vi "Close Library.vi"(8 "error in (no error)":errorcluster, 11 "library":refnum<vi>) -> (0 "error out":errorcluster)   [LabVIEW 2017, in "WebServiceImporter.lvlib" / "VI Generator.lvlib"]
uses:
  <vilib>/Platform/WebService/VI Generator/VI Generator.lvlib
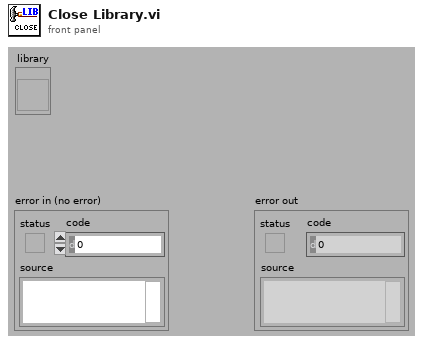
[diagram p1: front panel]
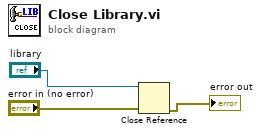
[diagram p0: block diagram]
diagram:
  n1 = Close Reference(reference="library", error in (no error)="error in (no error)") -> (error out=→"error out":errorcluster)
